vi "Deinitialize SPI.vi"(11 "Tasks in":T1) -> (0 "error out":errorcluster)   [LabVIEW 2023, in "SPI.lvlib"]
uses:
  SPI.lvlib
  Tasks.ctl
  <vilib>/DAQmx/write.llb/DAQmx Write (Digital Bool 1Line 1Point).vi
  <vilib>/DAQmx/miscellaneous.llb/DAQmx Fill In Error Info.vi
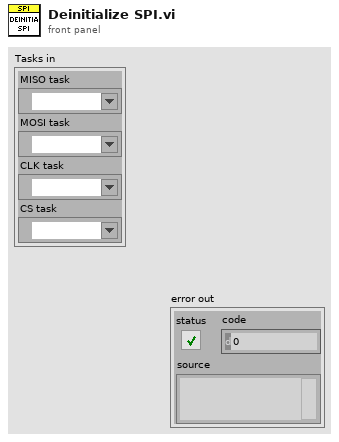
[diagram p1: front panel]
types:
  T1 = typedef "SPI.lvlib/Tasks.ctl" = cluster{"MISO task":refnum<k21>, "MOSI task":refnum<k21>, "CLK task":refnum<k21>, "CS task":refnum<k21>}
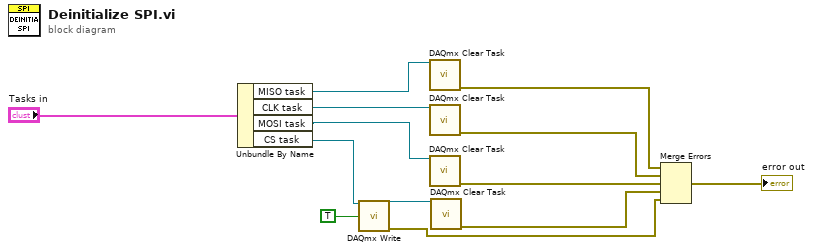
[diagram p0: block diagram]
diagram:
  n1 = Unbundle By Name("Tasks in") -> ("MISO task"=w7:refnum<k21>, "CLK task"=w8:refnum<k21>, "MOSI task"=w9:refnum<k21>, "CS task"=w10:refnum<k21>)
  n2 = call-poly <vilib>:"DAQmx Write.vi"("task/channels in"=w10, "data"=TRUE) -> ("task out"=w4:refnum<k21>, "error out"=w13:errorcluster)  [unwired: 11 in, 1 out]
  n3 = call <vilib>:"DAQmx Clear Task.vi"("task in"=w7) -> ("error out"=w1:errorcluster)  [unwired: 14 in]
  n4 = call <vilib>:"DAQmx Clear Task.vi"("task in"=w8) -> ("error out"=w2:errorcluster)  [unwired: 14 in]
  n5 = call <vilib>:"DAQmx Clear Task.vi"("task in"=w9) -> ("error out"=w3:errorcluster)  [unwired: 14 in]
  n6 = call <vilib>:"DAQmx Clear Task.vi"("task in"=w4) -> ("error out"=w11:errorcluster)  [unwired: 14 in]
  n7 = Merge Errors(w1, w2, w3, w11, w13) -> (→"error out":errorcluster)
